vi "ProcessDigitalOutput.vi"(11 "MockDigitalOutput":cluster{"BufferUpdateFIFO":refnum<k21>}={"BufferUpdateFIFO"="MockDigitalOutputCommand"}) -> ()   [LabVIEW 2016, in "FPGAMockDigitalOutput.lvlib"]
uses:
  FPGAMockDigitalOutput.lvlib
  <vilib>/rvi/Emulation/niFpgaGetClockAttributes.vi
  <vilib>/rvi/Emulation/niFpgaSctlEmulationGetInTimedLoop.vi
  <vilib>/rvi/Emulation/niFpgaEmulationReportErrorSimple.vi
  <vilib>/rvi/Emulation/niFpgaCriticalErrorInLSC.vi
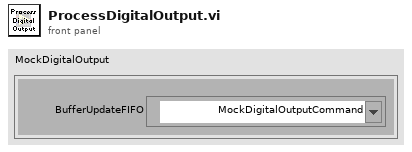
[diagram p1: front panel]
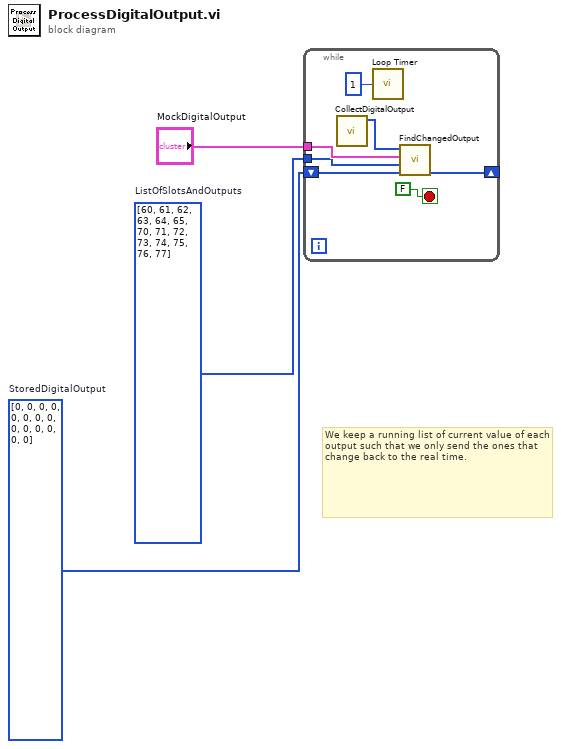
[diagram p0: block diagram]
diagram:
  w1 = u8[] [60, 61, 62, 63, 64, 65, 70, 71, 72, 73, 74, 75, 76, 77]  # ListOfSlotsAndOutputs
  w2 = u8[] [0, 0, 0, 0, 0, 0, 0, 0, 0, 0, 0, 0, 0, 0]  # StoredDigitalOutput
  # "We keep a running list of current value of each output such that we only send the ones that \nchange back to the real time."
  n1 = while {
    tunnel: "MockDigitalOutput" -> [w7]
    shift-right: [w4] -> _
    shift-left: w2 -> [w5]
    tunnel: w1 -> [w6]
    stop <- FALSE stop-if-true
    n2 = call "CollectDigitalOutput.vi"() -> ("U8 Array Out"=w8:u8[])  [unwired: 11 in]
    n3 = call "Loop Timer"("Count(uSec)"=u32 1 ("Count(mSec)")) -> ()  [unwired: 1 out]
    n4 = call "FindChangedOutput.vi"("StoredDigitalOutput"=w5, "ListOfSlotsAndOutputs"=w6, "MockDigitalOutput"=w7, "NewDigitalOutput"=w8) -> ("NewStoredDigitalOutput"=w4:u8[])  [unwired: 7 in]
  }
